vi "Write trigger holdoff (500.0 E-9 s).vi"(8 "error in (no error)":errorcluster, 10 "trigger holdoff (500.0 E-9 s)":dbl[unit]=5e-07 format="%^.2e", 11 "Configure Trigger Msg in":refnum<class "Configure Trigger Msg.lvclass">) -> (0 "error out":errorcluster, 3 "Configure Trigger Msg out":refnum<class "Configure Trigger Msg.lvclass">)   [LabVIEW 2016, in "CS++Scope.lvlib" / "Configure Trigger Msg.lvclass"]
uses:
  Configure Trigger Msg.lvclass
  Configure Trigger Msg.lvclass/Configure Trigger Msg.ctl
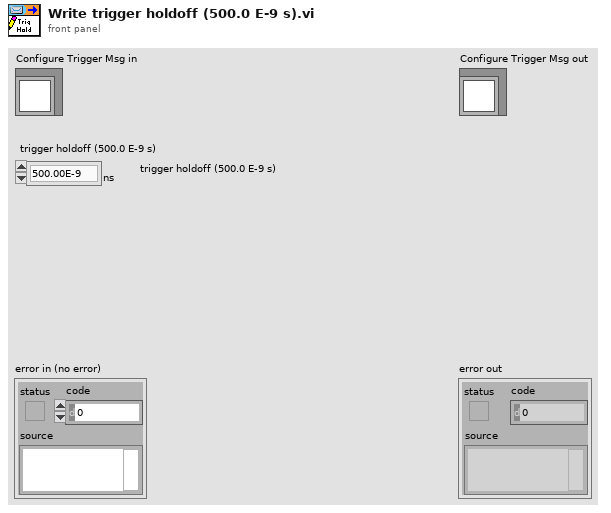
[diagram p1: front panel]
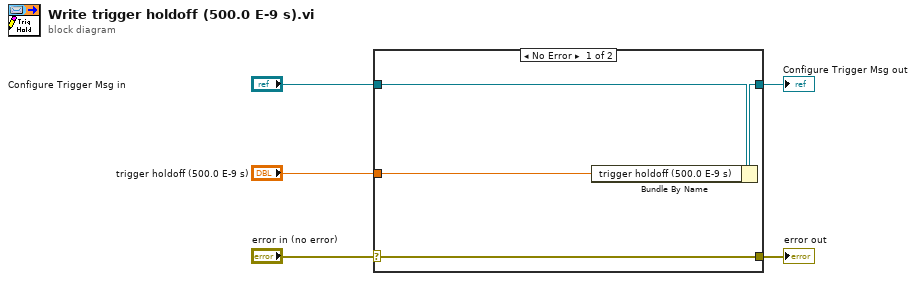
[diagram p0: block diagram]
diagram:
  n1 = case shown="No Error" "error in (no error)" {
    selector: "error in (no error)" -> [w9 w10]
    tunnel: [w9 w10] -> w4
    tunnel: [w7 w11] -> w2
    tunnel: "Configure Trigger Msg in" -> [w8 w11]
    tunnel: "trigger holdoff (500.0 E-9 s)" -> [w6 _]
    frame No Error {
      n2 = Bundle By Name(cluster=w8, "trigger holdoff (500.0 E-9 s)"=w6) -> (w7:refnum<class "Configure Trigger Msg.lvclass">)
    }
    frame Error {
    }
  }
  "error out" <- w4
  "Configure Trigger Msg out" <- w2
